vi "SineWaveform.vi"() -> ()   [LabVIEW 2020]
uses:
  <vilib>/measure/maUtilsandCtls.llb/ma_Updatet0 timestamp.vi
  <vilib>/measure/NI_MABase.lvlib
  <vilib>/Analysis/NI_AALBase.lvlib
panel:
  out "signal out":waveform(dbl)
  in  "offset":dbl format="%0.2p"
  in  "amplitude":dbl=1.0 format="%0.2p"
  in  "phase":dbl format="%.2p"
  in  "reset signal":bool
  in  "sampling info":cluster{"Fs":dbl, "#s":dbl}={"Fs"=1000.0, "#s"=1000.0} {"Fs" format="%.2p"}
  in  "frequency":dbl=10.0 format="%0.2p"
  out "error out":errorcluster
  in  "error in (no error)":errorcluster
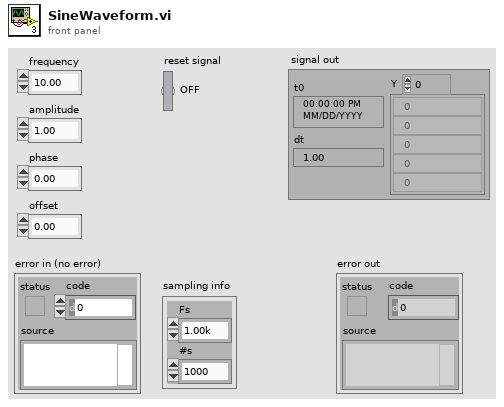
[diagram p1: front panel]
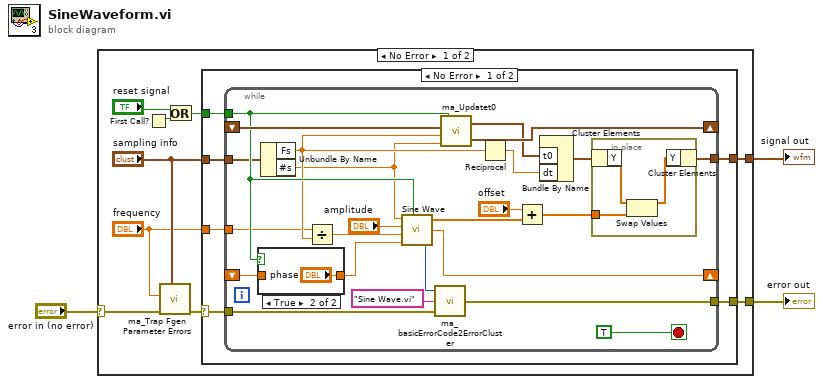
[diagram p0: block diagram]
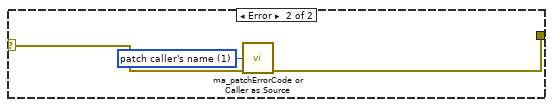
[diagram p3: hidden frame]
diagram:
  n1 = case shown="No Error" "error in (no error)" {
    selector: "error in (no error)" -> [w5 w51]
    tunnel: [w6 w51] -> w3
    tunnel: [w4 _] -> w1
    frame No Error {
      n2 = First Call?() -> (First Call?: T/F=w10:bool)
      n3 = call <vilib>:"ma_Trap Fgen Parameter Errors.vi"("Sampling info"="sampling info", "error in (no error)"=w5, "frequency"="frequency") -> ("error out"=w9:errorcluster)  [unwired: 8 in]
      n4 = Or(x="reset signal", y=w10) -> (x .or. y?=w11:bool)
      n5 = case shown="No Error" w9 {
        selector: w9 -> [w14 w50]
        tunnel: w11 -> [w18 _]
        tunnel: "sampling info" -> [w17 _]
        tunnel: "frequency" -> [w16 _]
        tunnel: [w15 w49] -> w6
        tunnel: [w13 _] -> w4
        frame No Error {
          n6 = while {
            tunnel: w14 -> [w24]
            tunnel: [w25] -> w15
            tunnel: w16 -> [w26]
            tunnel: w17 -> [w27]
            tunnel: w18 -> [w31]
            shift-left: _ -> [w33]
            shift-right: [w35] -> _
            shift-left: _ -> [w39]
            shift-right: [w38] -> _
            tunnel: [w19] -> w13
            stop <- TRUE stop-if-true
            n7 = case shown="True" w31 {
              tunnel: [w46 "phase"] -> w34
              tunnel: w33 -> [w46 _]
              frame False {
              }
              frame True {
              }
            }
            n8 = Unbundle By Name(w27) -> ("Fs"=w29:dbl, "#s"=w28:dbl)
            n9 = Divide(x=w26, y=w29) -> (x/y=w30:dbl)
            n10 = call <vilib>:"Sine Wave.vi"("samples"=w28, "amplitude"="amplitude", "frequency"=w30, "phase in"=w34, "reset phase"=w31) -> ("sine wave"=w36:dbl[], "phase out"=w35:dbl, "error"=w42:i32)
            n11 = call <vilib>:"ma_basicErrorCode2ErrorCluster.vi"("error in (no error)"=w24, "subVI name"="Sine Wave.vi" ("subVI Name"), "Error Code"=w42) -> ("error out"=w25:errorcluster)
            n12 = call-poly <vilib>:"ma_Updatet0.vi"("samples"=w28, "sampling rate (S/s)"=w29, "tf previous"=w39, "Reset Generation"=w31) -> ("tf new"=w38:timestamp, "t0"=w22:timestamp)
            n13 = Reciprocal(x=w29) -> (1/x=w23:dbl)
            n14 = Add(x="offset", y=w36) -> (x+y=w20:dbl[])
            n15 = Bundle By Name("t0"=w22, "dt"=w23) -> (w21:waveform(dbl))  [unwired: 1 in]
            n16 = in-place {
              in-place-border: w20 -> [w43]
              n17 = in-place-cluster #1(w21) -> ("Y"=w45:dbl[])
              n18 = Swap Values(12:w45, 14:w43) -> (1:w44:dbl[])  [unwired: 1 in, 1 out]
              n19 = in-place-cluster #1("Y"=w44) -> (w19:waveform(dbl))
            }
          }
        }
        frame Error {
          w48 = u16 1 items=["patch error code", "patch caller's name"] ("operation")
          n20 = call <vilib>:"ma_patchErrorCode or Caller as Source.vi"("error in (no error)"=w50, "operation"=w48) -> ("error out"=w49:errorcluster)  [unwired: 9 in]
        }
      }
    }
    frame Error {
    }
  }
  "error out" <- w3
  "signal out" <- w1
